vi "Run.vi"(8 "error in (no error)":errorcluster, 10 "TestResult":refnum<class "TestResult.lvclass">, 11 "TestSuite in":refnum<class "TestSuite.lvclass">) -> (0 "error out":errorcluster, 2 "TestResult out":refnum<class "TestResult.lvclass">, 3 "TestSuite out":refnum<class "TestSuite.lvclass">)   [LabVIEW 2019, in "TestSuite.lvclass"]
doc: "Runs the tests and collects their result in a <B>TestResult</B> object."
uses:
  TestSuite.lvclass
  TestResult/TestResult.lvclass
  TestSuite.lvclass/TestSuite.ctl
  Test/Test.lvclass
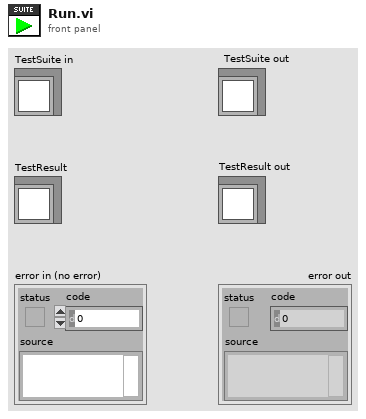
[diagram p1: front panel]
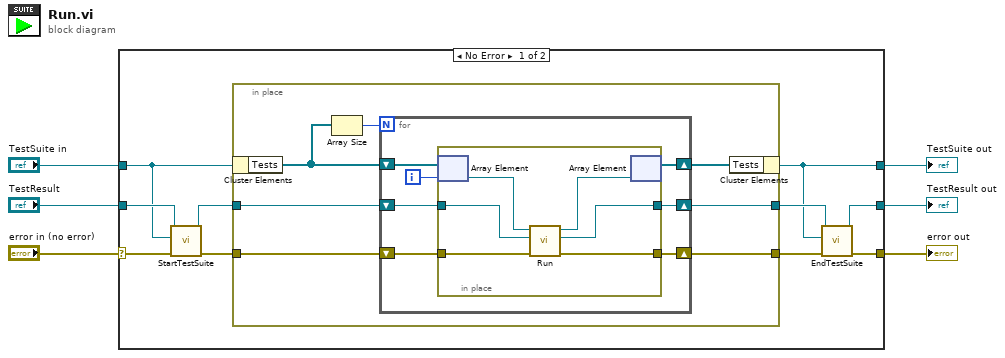
[diagram p0: block diagram]
diagram:
  n1 = case shown="No Error" "error in (no error)" {
    selector: "error in (no error)" -> [w15 w39]
    tunnel: "TestResult" -> [w14 w38]
    tunnel: [w11 w38] -> w5
    tunnel: [w13 w39] -> w4
    tunnel: "TestSuite in" -> [w9 w37]
    tunnel: [w10 w37] -> w1
    frame No Error {
      n2 = call-dynamic "StartTestSuite.vi"("error in (no error)"=w15, "TestSuite"=w9, "TestResult in"=w14) -> ("error out"=w7:errorcluster, "TestResult out"=w8:refnum<class "TestResult.lvclass">)  [unwired: 7 in]
      n3 = in-place {
        in-place-border: w8 -> [w23]
        in-place-border: [w22] -> w12
        in-place-border: [w21] -> w16
        in-place-border: w7 -> [w20]
        n4 = in-place-cluster #1(w9) -> ("Tests"=w18:refnum<class "Test.lvclass">[])
        n5 = Array Size(array=w18) -> (size(s)=w19:i32)
        n6 = for {
          N: w19 -> [_]
          shift-right: [w29] -> w22
          shift-left: w23 -> [w30]
          shift-right: [w28] -> w21
          shift-left: w20 -> [w27]
          shift-right: [w24] -> w17
          shift-left: w18 -> [w26]
          i -> [w25]
          n7 = in-place {
            in-place-border: w30 -> [w36]
            in-place-border: [w35] -> w29
            in-place-border: [w34] -> w28
            in-place-border: w27 -> [w33]
            n8 = in-place-array #2(w26, w25) -> (w32:refnum<class "Test.lvclass">)
            n9 = call-dynamic "Run.vi"("error in (no error)"=w33, "TestResult"=w36, "Test In"=w32) -> ("error out"=w34:errorcluster, "TestResult out"=w35:refnum<class "TestResult.lvclass">, "Test Out"=w31:refnum<class "Test.lvclass">)  [unwired: 6 in]
            n10 = in-place-array #2(w31) -> (w24:refnum<class "Test.lvclass">[])  [unwired: 1 out]
          }
        }
        n11 = in-place-cluster #1("Tests"=w17) -> (w10:refnum<class "TestSuite.lvclass">)
      }
      n12 = call-dynamic "EndTestSuite.vi"("error in (no error)"=w16, "TestSuite"=w10, "TestResult in"=w12) -> ("error out"=w13:errorcluster, "TestResult out"=w11:refnum<class "TestResult.lvclass">)  [unwired: 7 in]
    }
    frame Error {
    }
  }
  "error out" <- w4
  "TestSuite out" <- w1
  "TestResult out" <- w5
